vi "Populate Past Config Listbox.vi"(8 "error in (no error)":errorcluster, 11 "Refnum in":T1) -> (0 "error out":errorcluster, 2 "Past Configs Array":string[](array[string]), 3 "Refnum out":T1)   [LabVIEW 2017]
uses:
  <vilib>/Utility/config.llb/Config Data RefNum.ctl
  <vilib>/Utility/config.llb/Read Key (String).vi
  <vilib>/Utility/config.llb/NI_LVConfig.lvlib
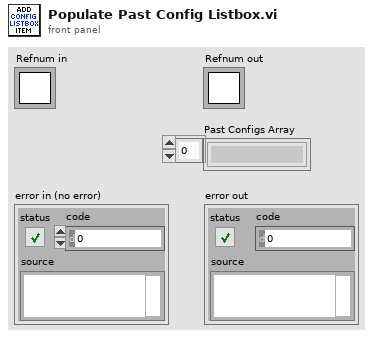
[diagram p1: front panel]
types:
  T1 = typedef "NI_LVConfig.lvlib/Config Data RefNum.ctl" = refnum<k1>
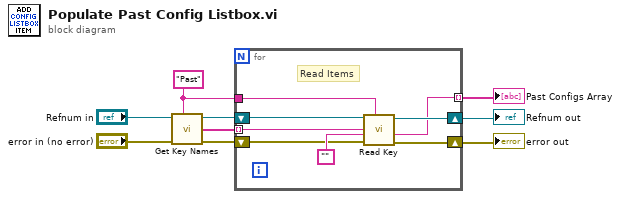
[diagram p0: block diagram]
diagram:
  w2 = "Past" ("section")
  n1 = call <vilib>:"Get Key Names.vi"("section"=w2, "error in (no error)"="error in (no error)", "refnum"="Refnum in") -> ("error out"=w3:errorcluster, "key names"=w1:string[], "refnum out"=w5:T1)  [unwired: 5 in, 1 out]
  n2 = for {
    shift-right: [w16] -> w8
    shift-left: w3 -> [w12]
    shift-right: [w15] -> w9
    shift-left: w5 -> [w13]
    tunnel: [w14] -> w7 mode=indexing
    tunnel: w2 -> [w11]
    tunnel: w1 -> [w10] mode=indexing
    # "Read Items"
    n3 = call-poly <vilib>:"Read Key.vi"("section"=w11, "error in (no error)"=w12, "default value"="", "key"=w10, "refnum"=w13) -> ("error out"=w16:errorcluster, "value"=w14:string, "refnum out"=w15:T1)  [unwired: 3 in, 1 out]
  }
  "Refnum out" <- w9
  "error out" <- w8
  "Past Configs Array" <- w7
